vi "Temperature_measurement.vi"() -> ()   [LabVIEW 2015]
panel:
  in  "VISA resource name 2":refnum<visa-resource-name>
  in  "VISA resource name":refnum<visa-resource-name>
  out "XY Graph":cluster{dbl[], dbl[]}(graph)
  in  "stop":bool
  in  "milliseconds to wait":u32
  out "number":dbl
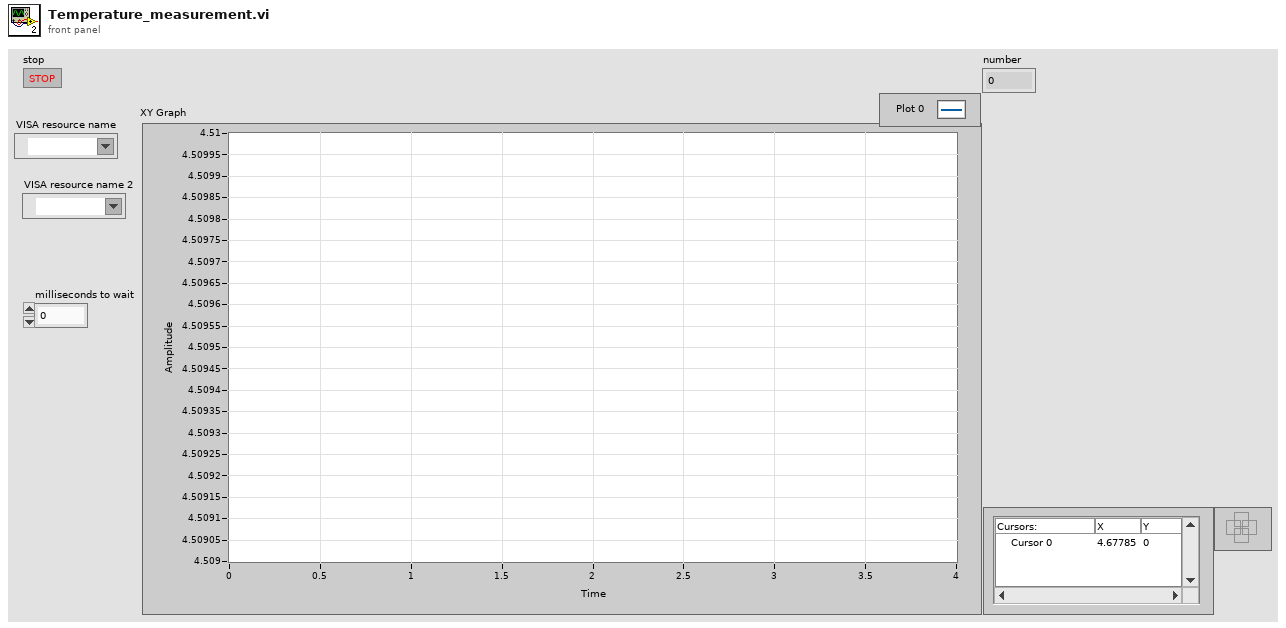
[diagram p1: front panel]
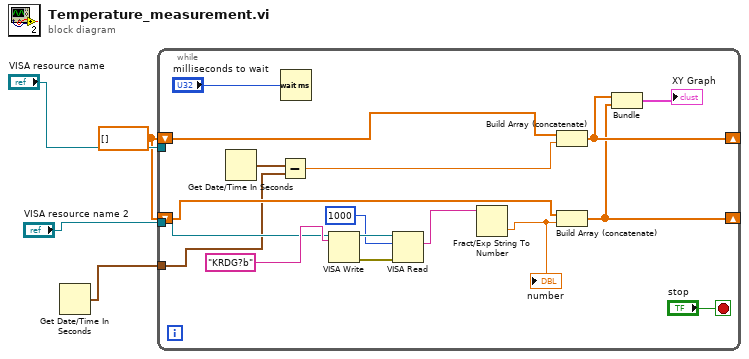
[diagram p0: block diagram]
diagram:
  w2 = dbl[] []
  n1 = Get Date/Time In Seconds() -> (seconds since 1Jan1904=w1:timestamp)
  n2 = while {
    tunnel: "VISA resource name" -> [_]
    tunnel: "VISA resource name 2" -> [w17]
    shift-right: [w5] -> _
    shift-left: w2 -> [w14]
    shift-right: [w6] -> _
    shift-left: w2 -> [w13]
    tunnel: w1 -> [w9]
    stop <- "stop" stop-if-true
    n3 = Get Date/Time In Seconds() -> (seconds since 1Jan1904=w10:timestamp)
    n4 = Subtract(x=w10, y=w9) -> (x-y=w8:dbl)
    n5 = Wait (ms)(milliseconds to wait="milliseconds to wait") -> ()  [unwired: 1 out]
    n6 = VISA Write(VISA resource name=w17, write buffer="KRDG?b") -> (VISA resource name out=w18:refnum<visa-resource-name>, error out=w20:errorcluster)  [unwired: 1 in, 1 out]
    n7 = VISA Read(VISA resource name=w18, byte count=u32 1000, error in (no error)=w20) -> (read buffer=w16:string)  [unwired: 3 out]
    n8 = Fract/Exp String To Number(string=w16) -> (number=w15:dbl)  [unwired: 3 in, 1 out]
    "number" <- w15
    n9 = Build Array (concatenate)(w13, w8) -> (w6:dbl[])
    n10 = Build Array (concatenate)(w14, w15) -> (w5:dbl[])
    n11 = Bundle(w6, w5) -> (→"XY Graph":cluster{dbl[], dbl[]})  [unwired: 1 in]
  }
